vi "Timer_GetAndReset.vi"(11 "In Timer":T1 {"Accumulated TIme" format="%13.5p"; "StartTime" format="%13.5p"}) -> (1 "CurrentTImer":dbl, 3 "out TIMER":T1 {"Accumulated TIme" format="%13.5p"; "StartTime" format="%13.5p"})   [LabVIEW 2019, in "Trajectory_Library.lvlib"]
doc: "Synchronized call to get and reset the timer. Get the current time from the timer. If the clock is running it is derived from the current system clock the start time stored in the timer class. If the clock is not running, then return the time when it was last stopped. Also reset the timer by setting the time to 0. Make the timer startTime the current time so new requests will be relative now.\n\nInputs:\n - Timer -- The Timer data cluster\n\nOutputs:\n - Timer -- The modified Timer data cluster\n - CurrentTimer -- Current time value for this timer in seconds"
uses:
  Trajectory_Library.lvlib
  TIMER.ctl
  Util_GetTime.vi
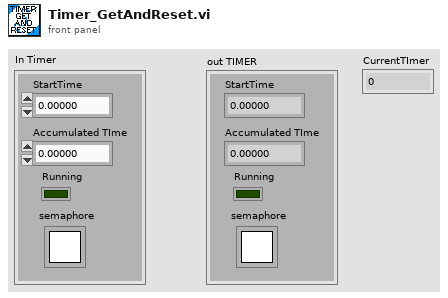
[diagram p1: front panel]
types:
  T1 = typedef "Trajectory_Library.lvlib/TIMER.ctl" = cluster{"StartTime":dbl, "Accumulated TIme":dbl, "Running":bool, "semaphore":T2}
  T2 = typedef "Semaphore RefNum" = refnum<k1>
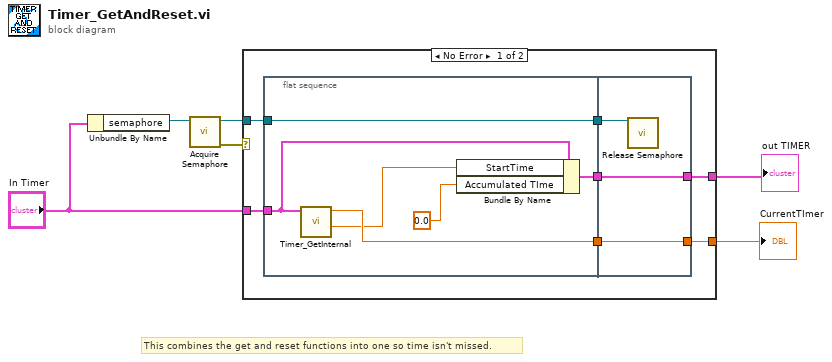
[diagram p0: block diagram]
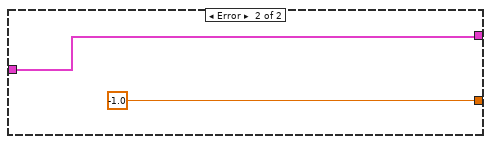
[diagram p2: hidden frame]
diagram:
  # "This combines the get and reset functions into one so time isn't missed."
  n1 = Unbundle By Name("In Timer") -> ("semaphore"=w4:T2)
  n2 = call <vilib>:"Acquire Semaphore.vi"("semaphore"=w4) -> ("error out"=w3:errorcluster, "semaphore out"=w2:T2)  [unwired: 4 in, 1 out]
  n3 = case shown="No Error" w3 {
    tunnel: [w13 -1.0 ("Accumulated TIme")] -> w6
    tunnel: "In Timer" -> [w12 w23]
    tunnel: w2 -> [w7 _]
    tunnel: [w11 w23] -> w1
    frame No Error {
      n4 = flat-sequence {
        tunnel: w12 -> [w18]
        tunnel: [w19] -> w10
        tunnel: [w15] -> w9
        tunnel: [w14] -> w8
        tunnel: w7 -> [w14]
        tunnel: [w21] -> w11
        tunnel: [w22] -> w13
        tunnel: w10 -> [w22]
        tunnel: w9 -> [w21]
        tunnel: w8 -> [w20]
        frame #0 {
          n5 = call "Timer_GetInternal.vi"("TIMER"=w18) -> ("SystemTime"=w16:dbl, "CurrentTImer"=w19:dbl)  [unwired: 9 in]
          n6 = Bundle By Name(cluster=w18, "StartTime"=w16, "Accumulated TIme"=0.0) -> (w15:T1)
        }
        frame #1 {
          n7 = call <vilib>:"Release Semaphore.vi"("semaphore"=w20) -> ()  [unwired: 5 in, 2 out]
        }
      }
    }
    frame Error {
    }
  }
  "CurrentTImer" <- w6
  "out TIMER" <- w1
